vi "Bold Description String.vi"(8 "error in (no error)":errorcluster, 9 "Selection":T1, 10 "String":string, 11 "String Ref":refnum<vi>) -> (0 "error out":errorcluster)   [LabVIEW 2023, in "VI Properties Editor.lvlib"]
doc: "Bolds a string with bold tags in it, modifying the selection to keep it the same as before."
uses:
  VI Properties Editor.lvlib
  <vilib>/Utility/miscctls.llb/LVSelectionTypeDef.ctl
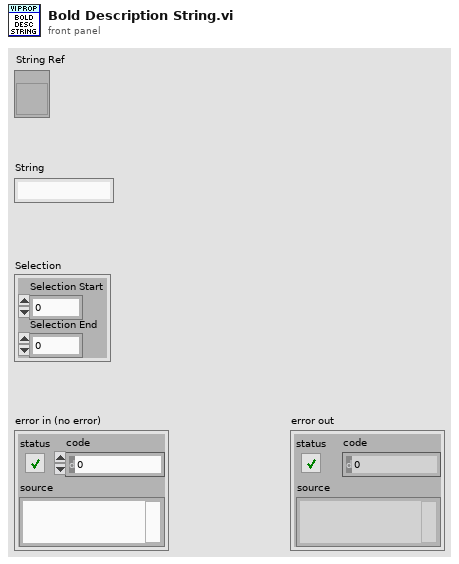
[diagram p1: front panel]
types:
  T1 = typedef "LVSelectionTypeDef.ctl" = cluster{"Selection Start":u32, "Selection End":u32}
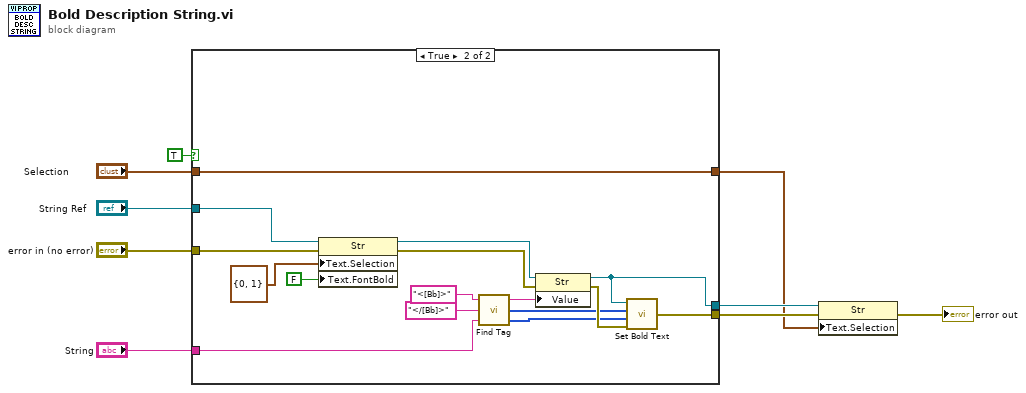
[diagram p0: block diagram]
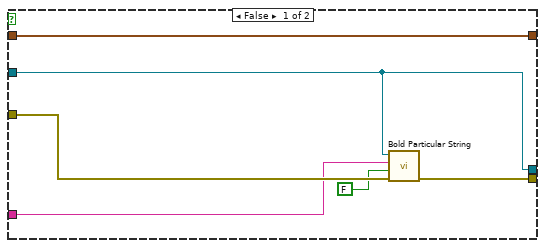
[diagram p2: hidden frame]
diagram:
  n1 = case shown="True" TRUE {
    tunnel: "error in (no error)" -> [w14 w30]
    tunnel: "String Ref" -> [w10 w29]
    tunnel: "String" -> [w13 w24]
    tunnel: [w11 w17] -> w5
    tunnel: [w10 w16] -> w4
    tunnel: [w15 w20] -> w3
    tunnel: "Selection" -> [w15 w20]
    frame False {
      n2 = call <vilib>:"Bold Particular String.vi"("error in (no error)"=w14, "resize string? (TRUE)"=FALSE, "text to display"=w13, "string refnum"=w10) -> ("error out"=w11:errorcluster)  [unwired: 6 in, 1 out]
    }
    frame True {
      n3 = property class="Str"(reference=w29, error in=w30, "Text.Selection"=T1 {"Selection Start"=0, "Selection End"=1}, "Text.FontBold"=FALSE ("Text.Font:Bold")) -> (reference out=w31:refnum<vi>, error out=w23:errorcluster)
      n4 = call <vilib>:"Find Tag.vi"("string"=w24, "close tag"="</[Bb]>", "open tag"="<[Bb]>") -> ("Length"=w21:i32[], "Start"=w22:i32[], "string out"=w26:string)
      n5 = property class="Str"(reference=w31, error in=w23, "Value"=w26) -> (reference out=w16:refnum<vi>, error out=w25:errorcluster)
      n6 = call <vilib>:"Set Bold Text.vi"("error in"=w25, "Length"=w21, "Start"=w22, "text"=w16) -> ("error out"=w17:errorcluster)  [unwired: 2 in]
    }
  }
  n7 = property class="Str"(reference=w4, error in=w5, "Text.Selection"=w3) -> (error out=→"error out":errorcluster)  [unwired: 1 out]
